vi "sendOutputData.vi"(8 "error in (no error)":errorcluster, 10 "outputData":T1 {"Step & Direction" min=-32767}, 11 "Context in":refnum<class "Context.lvclass">) -> (0 "error out":errorcluster, 3 "Context out":refnum<class "Context.lvclass">)   [LabVIEW 2013, in "Context.lvclass"]
uses:
  Context.lvclass
  <userlib>/Common/ILC/Typedefs/OutputData.ctl
  Context.lvclass/Context.ctl
  State/State.lvclass
  Model/Model/Model/Model.lvclass
  <userlib>/Common/ILC/Typedefs/ILCTypedefs.lvlib
panel:
  # "DAC"
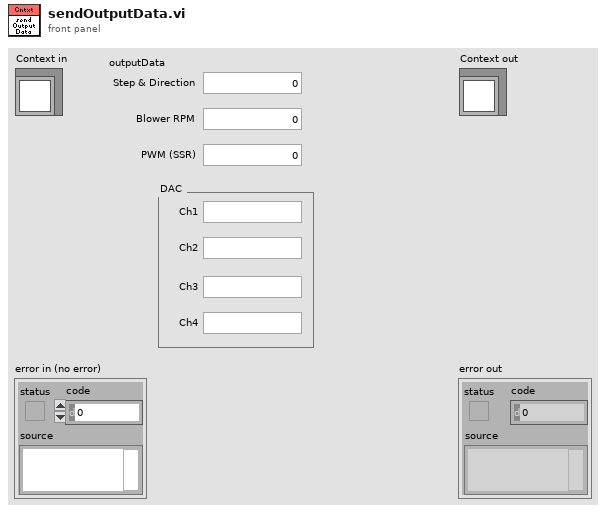
[diagram p1: front panel]
types:
  T1 = typedef "ILCCommon.lvlib/ILCTypedefs.lvlib/OutputData.ctl" = cluster{"Step & Direction":i16, "Blower RPM":u8, "PWM (SSR)":u8, "Ch1":u16, "Ch2":u16, "Ch3":u16, "Ch4":u16}
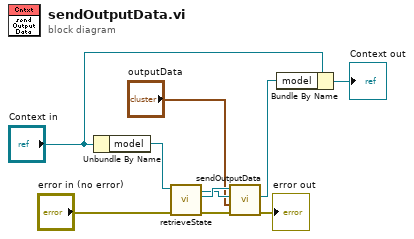
[diagram p0: block diagram]
diagram:
  n1 = Unbundle By Name("Context in") -> ("model"=w10:refnum<class "Model.lvclass">)
  n2 = call "retrieveState.vi"("error in (no error)"="error in (no error)", "Model in"=w10) -> ("error out"=w1:errorcluster, "state"=w7:refnum<class "State.lvclass">, "Model out"=w5:refnum<class "Model.lvclass">)  [unwired: 7 in]
  n3 = call-dynamic "sendOutputData.vi"("error in (no error)"=w1, "outputData"="outputData", "model"=w5, "State in"=w7) -> ("error out"=→"error out":errorcluster, "model 2"=w4:refnum<class "Model.lvclass">)  [unwired: 5 in, 1 out]
  n4 = Bundle By Name(cluster="Context in", "model"=w4) -> (→"Context out":refnum<class "Context.lvclass">)
